vi "Crosshairs.vi"(4 "MASTER in":T1 {"Image data"."Color Palette" items=["Grayscale U8", "False Color", "Overexposed"]; "Image data"."Exposure time [us]" format="%#_10g"; "Queue"."Initial time [s]" format="%_19f"; "Queue"."Raw data [V]\n(all samples)" format="%0.2f"; "Queue"."Timestamp [s]" format="%_19f"}) -> (1 "MASTER out":T1 {"Image data"."Color Palette" items=["Grayscale U8", "False Color", "Overexposed"]; "Image data"."Exposure time [us]" format="%#_10g"; "Queue"."Initial time [s]" format="%_19f"; "Queue"."Raw data [V]\n(all samples)" format="%0.2f"; "Queue"."Timestamp [s]" format="%_19f"})   [LabVIEW 2020]
uses:
  MASTER.ctl
  Constants.ctl
  QBundle.ctl
  Queue.ctl
  Image data.ctl
  <vilib>/userdefined/High Color/IMAQdx.ctl
  <vilib>/vision/Image Controls.llb/IMAQ Image.ctl
  Image QBundle.ctl
  <resource>/objmgr/imaqdx.rc
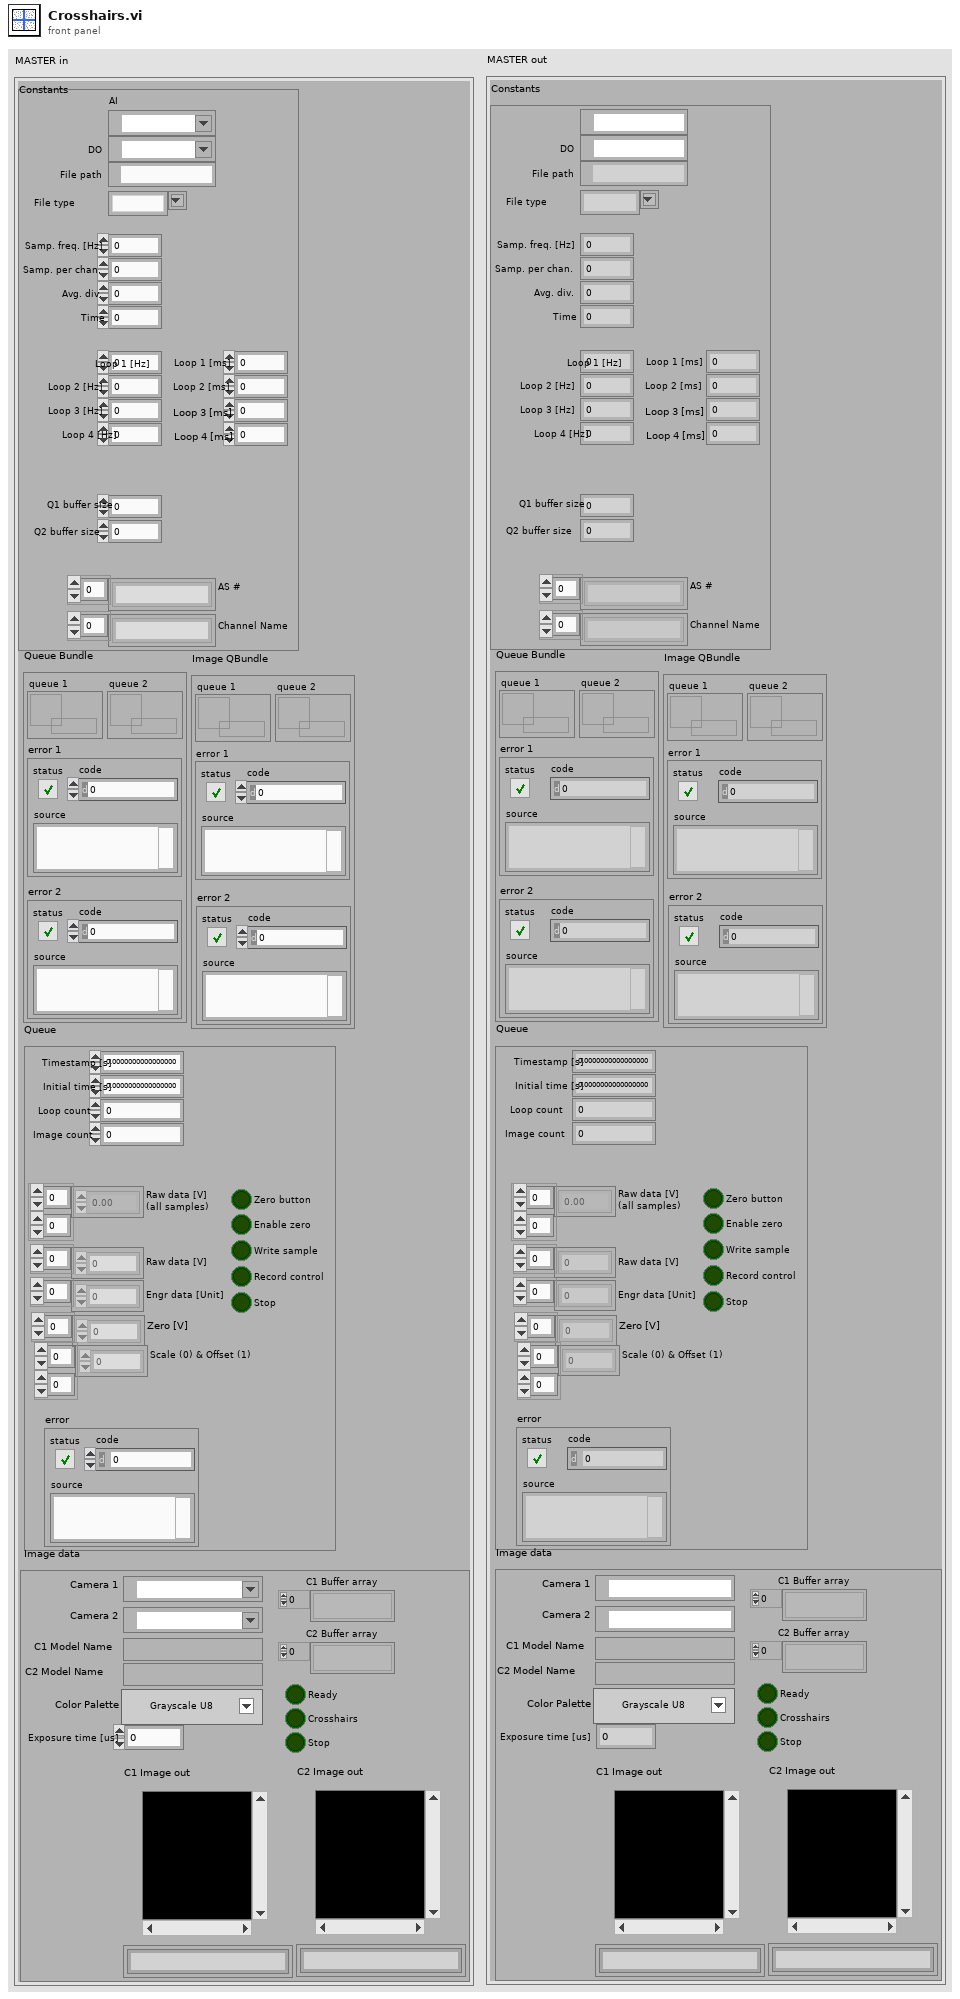
[diagram p1: front panel]
types:
  T1 = typedef "MASTER.ctl" = cluster{"Constants":T2, "Queue Bundle":T3, "Queue":T4, "Image data":T5, "Image QBundle ":T8}
  T2 = typedef "Constants.ctl" = cluster{"Time":u16, "Samp. freq. [Hz]":dbl, "Samp. per chan.":i32, "Avg. div.":i32, "File path":path, "AI":refnum<k21>, "Loop 1 [Hz]":dbl, "Loop 2 [Hz]":dbl, "Loop 3 [Hz]":dbl, "Loop 1 [ms]":dbl, "Loop 2 [ms]":dbl, "Loop 3 [ms]":dbl, "Q1 buffer size":i32, "Q2 buffer size":i32, "File type":string, "Loop 4 [Hz]":dbl, "Loop 4 [ms]":dbl, "Channel Name":string[], "AS #":string[], "DO":refnum<k21>}
  T3 = typedef "QBundle.ctl" = cluster{"queue 1":refnum<queue>, "error 1":errorcluster, "queue 2":refnum<queue>, "error 2":errorcluster}
  T4 = typedef "Queue.ctl" = cluster{"Enable zero":bool, "Engr data [Unit]":dbl[], "Zero button":bool, "Zero [V]":dbl[], "Timestamp [s]":dbl, "Write sample":bool, "Record control":bool, "Stop":bool, "error":errorcluster, "Raw data [V]\n(all samples)":dbl[][], "Raw data [V]":dbl[], "Loop count":i64, "Initial time [s]":dbl, "Scale (0) & Offset (1)":dbl[][], "Image count":dbl}
  T5 = typedef "Image data.ctl" = cluster{"Camera 1":T6, "Camera 2":T6, "C1 Image out ":T7, "C2 Image out":T7, "C1 Model Name":string, "C2 Model Name":string, "Exposure time [us]":dbl, "Color Palette":u16, "C1 Buffer array":T7[], "Ready":bool, "C2 Buffer array":T7[], "Crosshairs":bool, "Stop":bool}
  T6 = typedef "IMAQdx.ctl" = refnum<k21>
  T7 = typedef "IMAQ Image.ctl" = refnum<image>
  T8 = typedef "Image QBundle.ctl" = cluster{"queue 1":refnum<queue>, "error 1":errorcluster, "queue 2":refnum<queue>, "error 2":errorcluster}
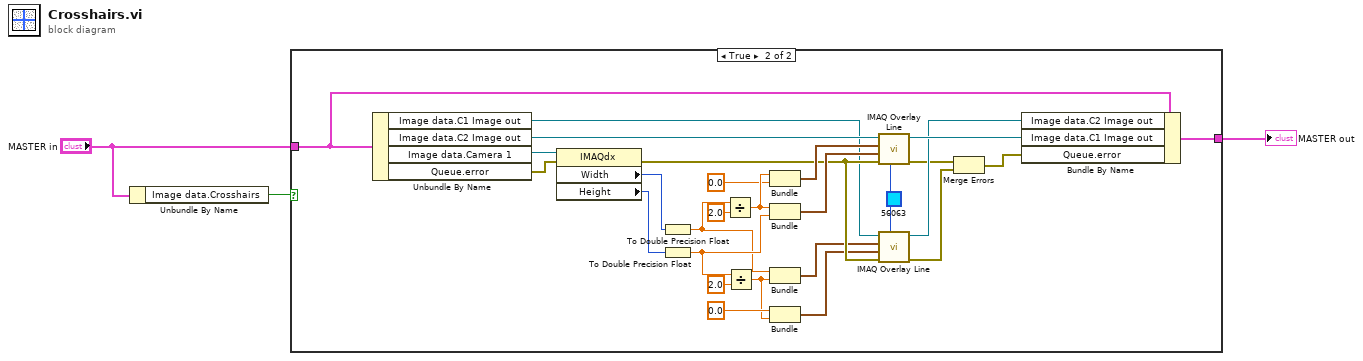
[diagram p0: block diagram]
diagram:
  n1 = Unbundle By Name("MASTER in") -> ("Image data.Crosshairs"=w1:bool)
  n2 = case shown="True" w1 {
    tunnel: "MASTER in" -> [w4 w31]
    tunnel: [w4 w30] -> w3
    frame False {
    }
    frame True {
      w9 = u32 56063 ("Color")
      n3 = Unbundle By Name(w31) -> ("Image data.C1 Image out"=w10:T7, "Image data.C2 Image out"=w19:T7, "Image data.Camera 1"=w29:T6, "Queue.error"=w27:errorcluster)
      n4 = property class="IMAQdx"(reference=w29, error in=w27) -> (error out=w13:errorcluster, "Width"=w28:u32, "Height"=w22:u32)  [unwired: 1 out]
      n5 = To Double Precision Float(number=w28) -> (double precision float=w16:dbl)
      n6 = To Double Precision Float(number=w22) -> (double precision float=w17:dbl)
      n7 = Divide(x=w16, y=2.0) -> (x/y=w24:dbl)
      n8 = Divide(x=w17, y=2.0) -> (x/y=w14:dbl)
      n9 = Bundle(w24, "y"=0.0) -> (w21:cluster{dbl, "y":dbl})  [unwired: 1 in]
      n10 = Bundle(w24, w17) -> (w20:cluster{dbl, dbl})  [unwired: 1 in]
      n11 = Bundle(w16, w14) -> (w12:cluster{dbl, dbl})  [unwired: 1 in]
      n12 = Bundle("y"=0.0, w14) -> (w11:cluster{"y":dbl, dbl})  [unwired: 1 in]
      n13 = call "IMAQ Overlay Line"("Color"=w9, "error in (no error)"=w13, "End Point"=w20, "Start Point"=w21, "Image"=w19) -> ("error out"=w6:errorcluster, "Image Out"=w18:T7)  [unwired: 5 in]
      n14 = call "IMAQ Overlay Line"("Color"=w9, "error in (no error)"=w13, "End Point"=w11, "Start Point"=w12, "Image"=w10) -> ("error out"=w5:errorcluster, "Image Out"=w8:T7)  [unwired: 5 in]
      n15 = Merge Errors(w6, w5) -> (w7:errorcluster)
      n16 = Bundle By Name(cluster=w31, "Image data.C2 Image out"=w8, "Image data.C1 Image out"=w18, "Queue.error"=w7) -> (w30:T1)
    }
  }
  "MASTER out" <- w3
